vi "test_BuildAssetsIncrementalBuild.vi"() -> (0 "error out":errorcluster, 3 "Pass?":bool)   [LabVIEW 2019, in "Tests.SolutionBuilder.lvlib"]
uses:
  Tests.SolutionBuilder.lvlib
  SolutionBuilder/SolutionBuilder.lvclass
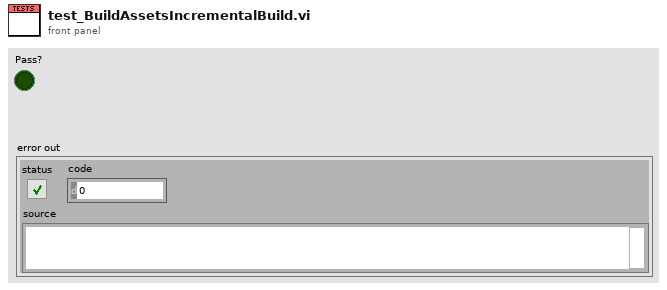
[diagram p1: front panel]
types:
  T1 = typedef "SolutionBuilder.lvlib/BuildManager.lvclass/GeneratedFile.ctl" = map{cluster{"Project path":string, "Build spec name":string}, set{string}}
  T2 = cluster{"Project path":string, "Build spec name":string}
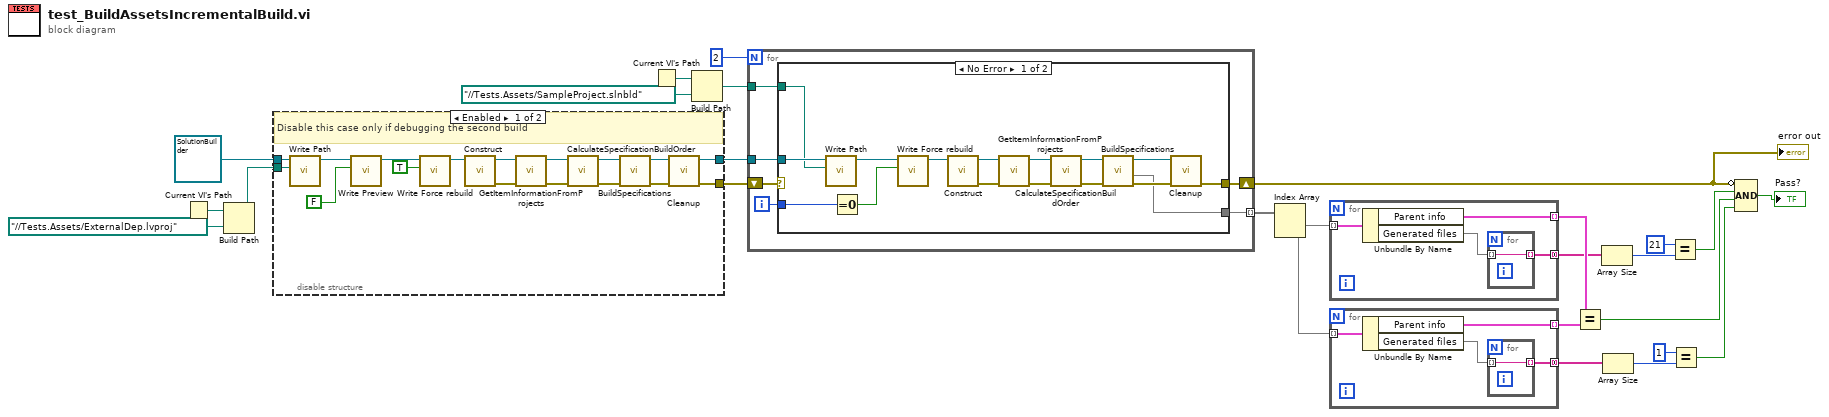
[diagram p0: block diagram]
diagram:
  n1 = Current VI's Path() -> (path=w24:path)
  n2 = Build Path(base path=w24, name or relative path=path "../../Tests.Assets/ExternalDep.lvproj" ("Path")) -> (appended path=w22:path)
  n3 = disable-structure shown="Enabled" {
    disable-tunnel: refnum<class "SolutionBuilder.lvclass"> refnum ("SolutionBuilder in") -> [w43 w44]
    disable-tunnel: w22 -> [w39 _]
    disable-tunnel: [w35 w44] -> w21
    disable-tunnel: [w33 _] -> w20
    frame Enabled {
      # "Disable this case only if debugging the second build"
      n4 = call "Write Path.vi"("Path"=w39, "SolutionBuilder in"=w43) -> ("SolutionBuilder out"=w31:refnum<class "SolutionBuilder.lvclass">)  [unwired: 9 in]
      n5 = call "Write Preview.vi"("Preview?"=FALSE, "SolutionBuilder in"=w31) -> ("SolutionBuilder out"=w29:refnum<class "SolutionBuilder.lvclass">)  [unwired: 9 in]
      n6 = call "Write Force rebuild.vi"("Force rebuild"=TRUE, "SolutionBuilder in"=w29) -> ("SolutionBuilder out"=w28:refnum<class "SolutionBuilder.lvclass">)  [unwired: 9 in]
      n7 = call "Construct.vi"("SolutionBuilder in"=w28) -> ("error out"=w38:errorcluster, "SolutionBuilder out"=w42:refnum<class "SolutionBuilder.lvclass">)  [unwired: 9 in]
      n8 = call "GetItemInformationFromProjects.vi"("error in (no error)"=w38, "SolutionBuilder in"=w42) -> ("error out"=w37:errorcluster, "SolutionBuilder out"=w41:refnum<class "SolutionBuilder.lvclass">)  [unwired: 8 in]
      n9 = call "CalculateSpecificationBuildOrder.vi"("error in (no error)"=w37, "SolutionBuilder in"=w41) -> ("error out"=w36:errorcluster, "SolutionBuilder out"=w40:refnum<class "SolutionBuilder.lvclass">)  [unwired: 8 in]
      n10 = call "BuildSpecifications.vi"("error in (no error)"=w36, "SolutionBuilder in"=w40) -> ("error out"=w34:errorcluster, "SolutionBuilder out"=w32:refnum<class "SolutionBuilder.lvclass">)  [unwired: 7 in, 1 out]
      n11 = call "Cleanup.vi"("error in (no error)"=w34, "SolutionBuilder in"=w32) -> ("error out"=w33:errorcluster, "SolutionBuilder out"=w35:refnum<class "SolutionBuilder.lvclass">)  [unwired: 8 in]
    }
    frame Disabled {
    }
  }
  n12 = Current VI's Path() -> (path=w19:path)
  n13 = Build Path(base path=w19, name or relative path=path "../../Tests.Assets/SampleProject.slnbld" ("Path")) -> (appended path=w17:path)
  n14 = for {
    N: 2 -> [_]
    tunnel: w21 -> [w49]
    tunnel: w17 -> [w47]
    shift-right: [w50] -> w26
    shift-left: w20 -> [w48]
    tunnel: [w46] -> w16 mode=indexing
    i -> [w45]
    n15 = case shown="No Error" w48 {
      selector: w48 -> [_ w67]
      tunnel: w49 -> [w60 _]
      tunnel: [w58 w67] -> w50
      tunnel: w47 -> [w57 _]
      tunnel: [w56 _] -> w46
      tunnel: w45 -> [w52 _]
      frame No Error {
        n16 = call "Write Path.vi"("Path"=w57, "SolutionBuilder in"=w60) -> ("SolutionBuilder out"=w54:refnum<class "SolutionBuilder.lvclass">)  [unwired: 9 in]
        n17 = Equal To 0?(x=w52) -> (x = 0?=w51:bool)
        n18 = call "Write Force rebuild.vi"("Force rebuild"=w51, "SolutionBuilder in"=w54) -> ("SolutionBuilder out"=w53:refnum<class "SolutionBuilder.lvclass">)  [unwired: 9 in]
        n19 = call "Construct.vi"("SolutionBuilder in"=w53) -> ("error out"=w64:errorcluster, "SolutionBuilder out"=w61:refnum<class "SolutionBuilder.lvclass">)  [unwired: 9 in]
        n20 = call "GetItemInformationFromProjects.vi"("error in (no error)"=w64, "SolutionBuilder in"=w61) -> ("error out"=w65:errorcluster, "SolutionBuilder out"=w62:refnum<class "SolutionBuilder.lvclass">)  [unwired: 8 in]
        n21 = call "CalculateSpecificationBuildOrder.vi"("error in (no error)"=w65, "SolutionBuilder in"=w62) -> ("error out"=w66:errorcluster, "SolutionBuilder out"=w63:refnum<class "SolutionBuilder.lvclass">)  [unwired: 8 in]
        n22 = call "BuildSpecifications.vi"("error in (no error)"=w66, "SolutionBuilder in"=w63) -> ("error out"=w59:errorcluster, "Generated file"=w56:T1, "SolutionBuilder out"=w55:refnum<class "SolutionBuilder.lvclass">)  [unwired: 7 in]
        n23 = call "Cleanup.vi"("error in (no error)"=w59, "SolutionBuilder in"=w55) -> ("error out"=w58:errorcluster)  [unwired: 8 in, 1 out]
      }
      frame Error {
      }
    }
  }
  "error out" <- w26
  n24 = Index Array(array=w16) -> (element #1=w15:T1, element #2=w14:T1)  [unwired: 2 in]
  n25 = for {
    tunnel: w15 -> [w71] mode=indexing
    tunnel: [w70] -> w13 mode=indexing
    tunnel: [w68] -> w10 mode=concatenating
    n26 = Unbundle By Name(w71) -> ("Parent info"=w70:T2, "Generated files"=w69:set{string})
    n27 = for {
      tunnel: w69 -> [w72] mode=indexing
      tunnel: [w72] -> w68 mode=indexing
    }
  }
  n28 = for {
    tunnel: w14 -> [w76] mode=indexing
    tunnel: [w75] -> w12 mode=indexing
    tunnel: [w73] -> w5 mode=concatenating
    n29 = Unbundle By Name(w76) -> ("Parent info"=w75:T2, "Generated files"=w74:set{string})
    n30 = for {
      tunnel: w74 -> [w77] mode=indexing
      tunnel: [w77] -> w73 mode=indexing
    }
  }
  n31 = Equal?(x=w13, y=w12) -> (x = y?=w3:bool)
  n32 = Array Size(array=w10) -> (size(s)=w9:i32)
  n33 = Array Size(array=w5) -> (size(s)=w6:i32)
  n34 = Equal?(x=21, y=w9) -> (x = y?=w4:bool)
  n35 = Equal?(x=1, y=w6) -> (x = y?=w2:bool)
  n36 = Compound Arithmetic op=AND(invert w26, w4, w3, w2) -> (→"Pass?":bool)
